vi "ssh_.vi"() -> ()   [LabVIEW 2022 SP3]
uses:
  <vilib>/net/SSH/Client/OpenSSH/OpenSSH Client.lvclass
  C:/Program Files/National Instruments/LabVIEW 2022/vi.lib/net/SSH/Client/Generic/Generic Client.lvclass
  <vilib>/net/SSH/NI_SSH.lvlib
  <vilib>/net/SSH/Client/PuTTY/PuTTY Client.lvclass
panel:
  out "return code":i32
  out "standard output 2":string
  out "standard output":string
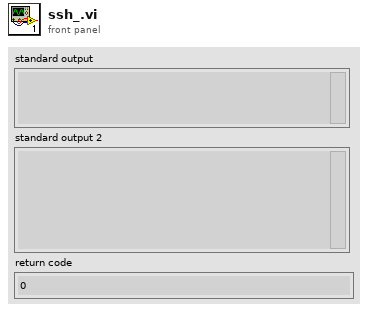
[diagram p1: front panel]
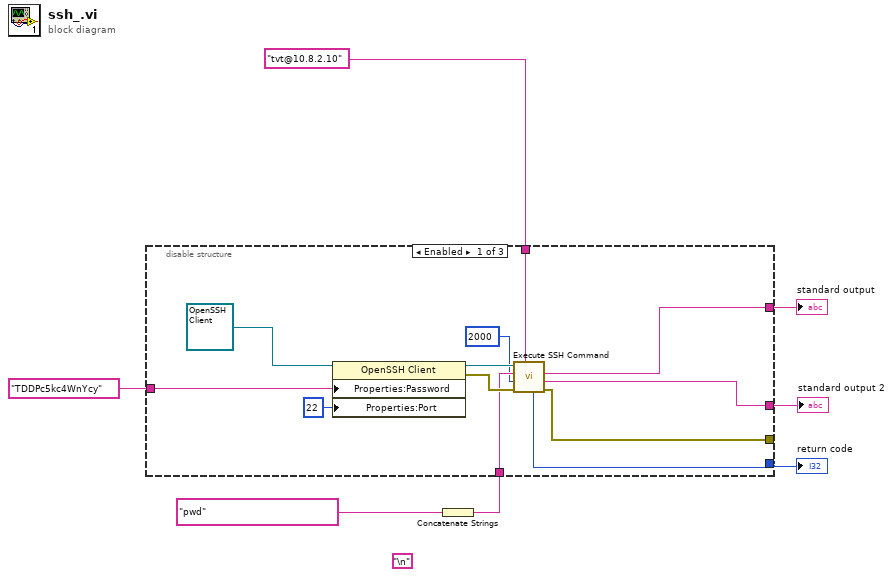
[diagram p0: block diagram]
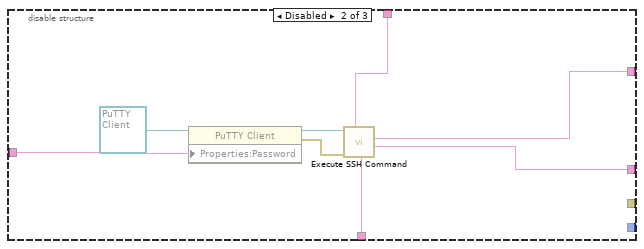
[diagram p2: hidden frame]
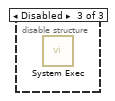
[diagram p3: hidden frame]
diagram:
  (unwired) "\n"
  n1 = Concatenate Strings("pwd" ("command line")) -> (w1:string)
  n2 = disable-structure shown="Enabled" {
    disable-tunnel: "tvt@10.8.2.10" ("user@host") -> [w16 w24 _]
    disable-tunnel: w1 -> [w15 w23 _]
    disable-tunnel: "TDDPc5kc4WnYcy" ("user@host") -> [w14 w22 _]
    disable-tunnel: [w13 w21 _] -> w4
    disable-tunnel: [w12 w20 _] -> w3
    disable-tunnel: [w11 _ _] -> _
    disable-tunnel: [w10 _ _] -> w2
    frame Enabled {
      n3 = property class="OpenSSH Client"(reference=refnum<class "OpenSSH Client.lvclass"> refnum ("NI_SSH.lvlib:OpenSSH Client"), "Properties:Password"=w14, "Properties:Port"=u16 22 ("Port")) -> (reference out=w18:refnum<class "OpenSSH Client.lvclass">, error out=w17:errorcluster)  [unwired: 1 in]
      n4 = call <vilib>:"Execute SSH Command.vi"("user@host"=w16, "error in (no error)"=w17, "timeout (ms)"=2000, "command line"=w15, "session in"=w18) -> ("error out"=w11:errorcluster, "standard error"=w12:string, "standard output"=w13:string, "return code"=w10:i32)  [unwired: 2 in, 1 out]
    }
    frame Disabled {
      n5 = property class="PuTTY Client"(reference=refnum<class "PuTTY Client.lvclass"> refnum ("NI_SSH.lvlib:PuTTY Client"), "Properties:Password"=w22) -> (reference out=w27:refnum<class "PuTTY Client.lvclass">, error out=w26:errorcluster)  [unwired: 1 in]
      n6 = call <vilib>:"Execute SSH Command.vi"("user@host"=w24, "error in (no error)"=w26, "command line"=w23, "session in"=w27) -> ("standard error"=w20:string, "standard output"=w21:string)  [unwired: 3 in, 3 out]
    }
    frame Disabled {
      n7 = call <vilib>:"System Exec.vi"() -> ()  [unwired: 8 in, 4 out]
    }
  }
  "standard output" <- w4
  "standard output 2" <- w3
  "return code" <- w2
